vi "Segment Log File (Footprint).vi"(8 "error in (no error)":errorcluster, 11 "Footprint Segmented Log in":refnum<class "Footprint Segmented Log.lvclass">) -> (0 "error out":errorcluster, 2 "Segment Log File":bool, 3 "Footprint Segmented Log out":refnum<class "Footprint Segmented Log.lvclass">)   [LabVIEW 2015, in "Footprint Segmented Log.lvclass"]
doc: "Segment the log file whenever the file reaches a specified max size in bytes. Checking the file size is slow and inaccurate due to buffering issues. Only do it after a minimum amount of time has elapsed."
uses:
  Footprint Segmented Log.lvclass
  Footprint Segmented Log.lvclass/Footprint Segmented Log.ctl
  Segmented Log/Segmented Log.lvclass/Segmented Log.ctl
  Log Files/Log File/Log File.lvclass/Log File.ctl
  Segmented Log/Segmented Log.lvclass
  Log Files/Log File/Log File.lvclass
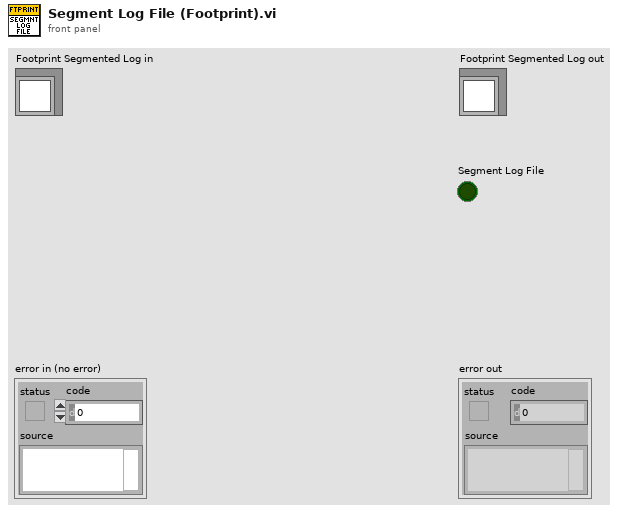
[diagram p1: front panel]
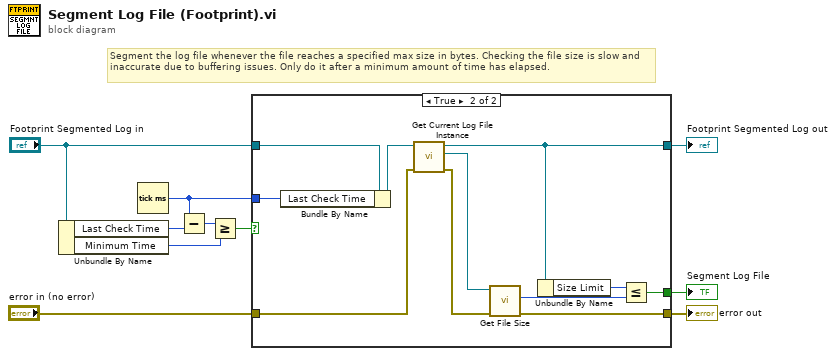
[diagram p0: block diagram]
diagram:
  # "Segment the log file whenever the file reaches a specified max size in bytes. Checking the file size is slow and inaccurate due to buffering issues. Only do it after a minimum amount of time has elapsed."
  n1 = Unbundle By Name("Footprint Segmented Log in") -> ("Last Check Time"=w6:u32, "Minimum Time"=w4:u32)
  n2 = Tick Count (ms)() -> (millisecond timer value=w1:u32)
  n3 = Subtract(x=w1, y=w6) -> (x-y=w5:u32)
  n4 = Greater Or Equal?(x=w5, y=w4) -> (x >= y?=w3:bool)
  n5 = case shown="True" w3 {
    tunnel: "error in (no error)" -> [w11 w23]
    tunnel: [w12 w18] -> w9
    tunnel: [_ w17] -> w8
    tunnel: [w11 w16] -> w7
    tunnel: "Footprint Segmented Log in" -> [w12 w15]
    tunnel: w1 -> [_ w13]
    frame False {
    }
    frame True {
      n6 = Bundle By Name(cluster=w15, "Last Check Time"=w13) -> (w14:refnum<class "Footprint Segmented Log.lvclass">)
      n7 = call "Get Current Log File Instance.vi"("error in (no error)"=w23, "Segmented Log in"=w14) -> ("error out"=w19:errorcluster, "Log File Instance"=w20:refnum<class "Log File.lvclass">, "Segmented Log out"=w18:refnum<class "Footprint Segmented Log.lvclass">)  [unwired: 7 in]
      n8 = call "Get File Size.vi"("error in (no error)"=w19, "Log File in"=w20) -> ("error out"=w16:errorcluster, "size (in bytes)"=w22:i64)  [unwired: 7 in, 1 out]
      n9 = Unbundle By Name(w18) -> ("Size Limit"=w21:i64)
      n10 = Less Or Equal?(x=w21, y=w22) -> (x <= y?=w17:bool)
    }
  }
  "error out" <- w7
  "Footprint Segmented Log out" <- w9
  "Segment Log File" <- w8
